vi "Actor Core.vi"(8 "Error In":errorcluster, 11 "KIT-QVG.lvclass":refnum<class "KIT-QVG.lvclass">) -> (0 "Error Out":errorcluster, 3 "Actor out":refnum<class "Actor.lvclass">)   [LabVIEW 2014, in "KIT-QVG.lvlib" / "KIT-QVG.lvclass"]
doc: "(<B>Filename</B>: Actor Framework.lvlib:Actor.lvclass:Actor Core.vi)\n\nReceives messages to the actor, reacts to them, and initiates any error handling that may shut the actor down.\n\nDescendant classes may override this VI to append parallel tasks for the actor to complete while it handles messages. Overrides use the Call Parent Method node."
uses:
  KIT-QVG.lvclass
  <vilib>/ActorFramework/Actor/Actor.lvclass
  CSPP_Core/Actors/CS++BaseActor/CS++BaseActor.lvclass/CS++BaseActor.ctl
  CSPP_Core/Actors/CS++GUIActor/CS++GUIActor.lvclass/CS++GUIActor.ctl
  CSPP_Core/Classes/CS++ProcessVariables/ProcessVariable/PV.lvclass/PV.ctl
  CSPP_Core/Classes/CS++ProcessVariables/PVConnection/PVConnection.lvclass/PVConnection.ctl
  <vilib>/ActorFramework/Actor/Actor.lvclass/Actor.ctl
  <vilib>/ActorFramework/Message Enqueuer/Message Enqueuer.lvclass/Message Enqueuer.ctl
  CSPP_Core/Actors/CS++BaseActor/Read Object Name.vi
  CSPP_Core/Actors/CS++BaseActor/Read CS++Factory.vi
  CSPP_Core/Actors/CS++GUIActor/Read Associated Actor Name.vi
  CSPP_Core/Actors/CS++GUIActor/Read Associated Proxy Actor Name.vi
  CSPP_Core/Classes/CS++ProcessVariables/ProcessVariable/Read Name.vi
  CSPP_Core/Classes/CS++ProcessVariables/ProcessVariable/Read Timestamp.vi
  CSPP_Core/Actors/CS++GUIActor/Read Stop-Event.vi
  CSPP_Core/Actors/CS++GUIActor/Read PV-Update.vi
  <vilib>/ActorFramework/Message Enqueuer/Init from Existing Queue.vi
  <vilib>/ActorFramework/Message Enqueuer/Enqueue.vi
  <vilib>/ActorFramework/Message Priority Queue/Priority Enqueue.vi
  CSPP_Core/Classes/CS++ProcessVariables/PVConnection/PVConnection.lvclass
  CSPP_Core/Classes/CS++BaseClasses/Factory/CS++Factory.lvclass
  CSPP_Core/Classes/CS++ProcessVariables/ProcessVariable/PV.lvclass
  <vilib>/ActorFramework/Message Enqueuer/Message Enqueuer.lvclass
  <vilib>/ActorFramework/Stop Msg/Stop Msg.lvclass
  CSPP_Core/Actors/CS++DeviceGUIActor/CS++DeviceGUIActor.lvclass
  CSPP_Core/Actors/CS++BaseActor/CS++BaseActor.lvclass
  CSPP_Core/Actors/CS++GUIActor/CS++GUIActor.lvclass
  CSPP_Core/Libraries/Utilities/CS++Utilities.lvlib
  CSPP_Core/Classes/CS++ProcessVariables/CS++ProcessVariables.lvlib
panel:
  out "Voltage":dbl[unit][](array[numeric]) format="%.4f"
  out "ADC Raw":i16[](array[numeric])
  out "Hardware Status":T1(array[cluster])
  out "Detector Status":T2(array[cluster])
  out "Temperature":dbl[unit]=273.15
  out "Rack Status":T3
  in  "Detector":u8
  in  "Mute":bool
  in  "Auto Mute":bool
  in  "Mute All":bool
  in  "Quench":bool
  in  "FQuit":bool
  in  "Stop":bool
  in  "Start":bool
  out "Associated Proxy Actor":string
  in  "Stop Button":bool
  out "Timestamp":timestamp
  out "Self-Test Result Message":string
  out "Self-Test Result Code":i32
  out "Resource Name":string
  out "Firmware Revision":string
  out "Driver Revision":string
  out "Associated Worker Actor":string
  # "Resize window to view more details."
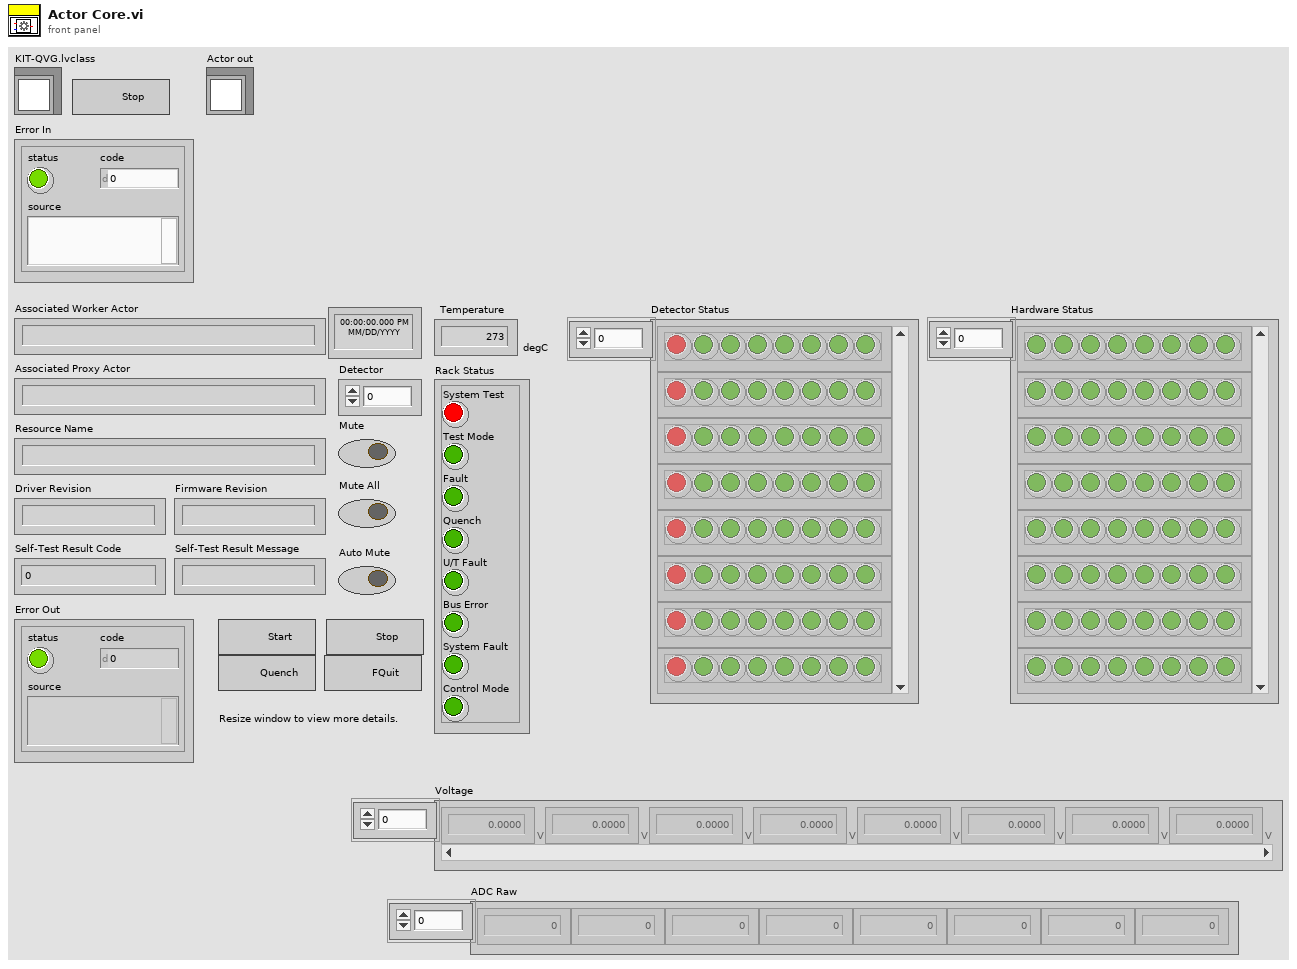
[diagram p1: front panel]
types:
  T1 = cluster{"Q1+":bool, "Q1-":bool, "Q2+":bool, "Q2-":bool, "Mute":bool, "STest-Bit":bool, "QD1":bool, "QD2":bool}[]
  T2 = cluster{"System Test":bool, "Test Mode":bool, "Fault":bool, "Quench":bool, "U/T Fault":bool, "Bus Error":bool, "System Fault":bool, "Reserved":bool}[]
  T3 = cluster{"System Test":bool, "Test Mode":bool, "Fault":bool, "Quench":bool, "U/T Fault":bool, "Bus Error":bool, "System Fault":bool, "Control Mode":bool}
  T4 = cluster{"Read Access":enum8{"Allowed", "Required", "None"}, "Write Access":enum8{"Allowed", "Required", "None"}}
  T5 = enum32{"Invalid", "Standard", "Closed", "Hidden", "Minimized", "Maximized"}
  T6 = cluster{"Q1+":bool, "Q1-":bool, "Q2+":bool, "Q2-":bool, "Mute":bool, "STest-Bit":bool, "QD1":bool, "QD2":bool}
  T7 = cluster{"System Test":bool, "Test Mode":bool, "Fault":bool, "Quench":bool, "U/T Fault":bool, "Bus Error":bool, "System Fault":bool, "Reserved":bool}
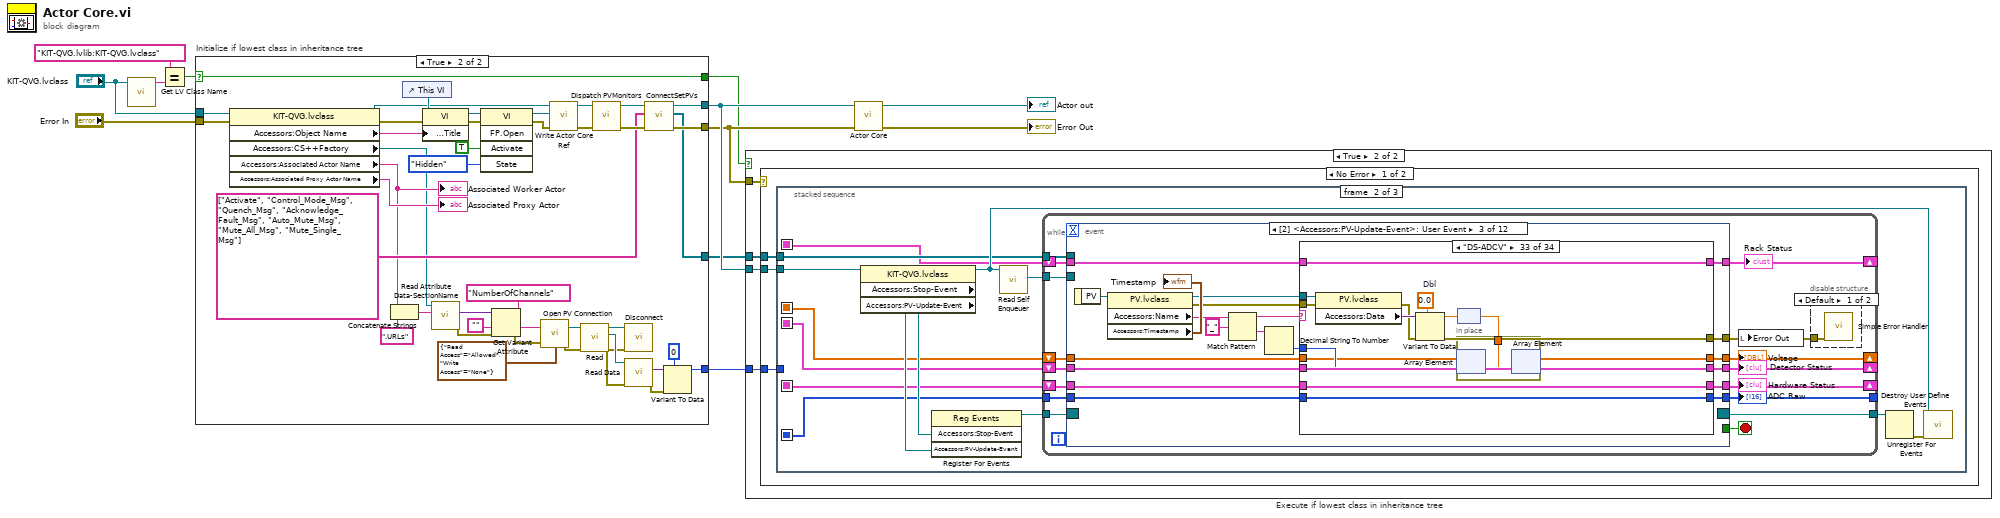
[diagram p0: block diagram]
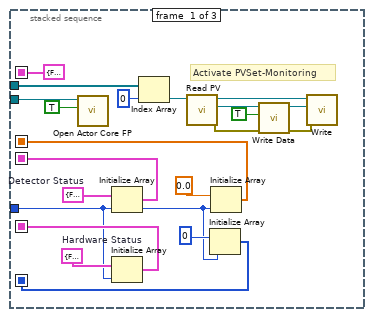
[diagram p3: hidden frame]
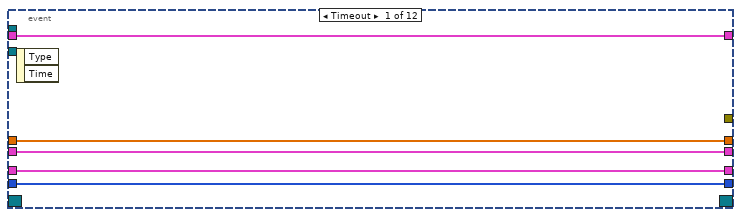
[diagram p5: hidden frame]
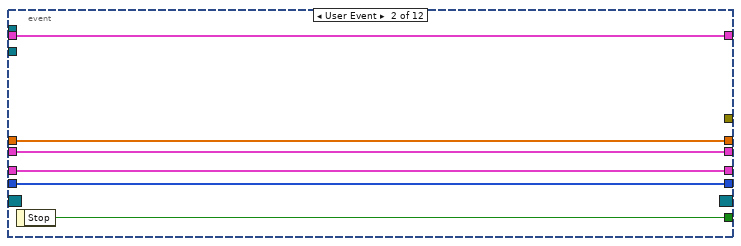
[diagram p6: hidden frame]
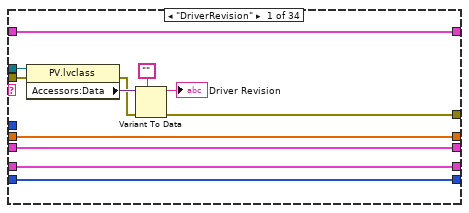
[diagram p7: hidden frame]
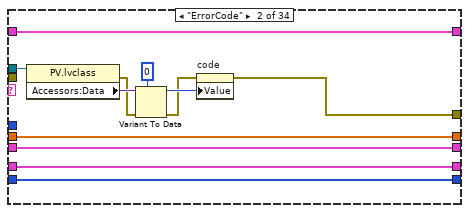
[diagram p8: hidden frame]
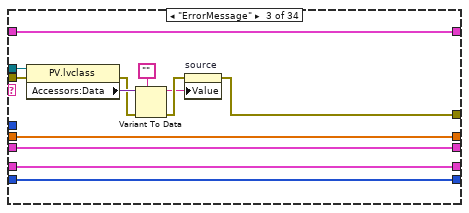
[diagram p9: hidden frame]
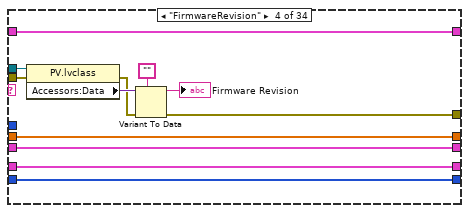
[diagram p10: hidden frame]
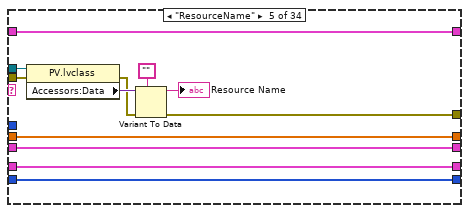
[diagram p11: hidden frame]
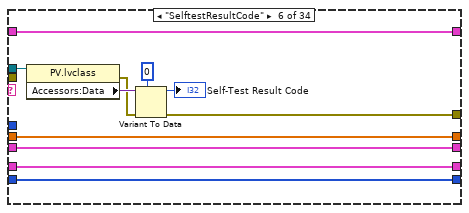
[diagram p12: hidden frame]
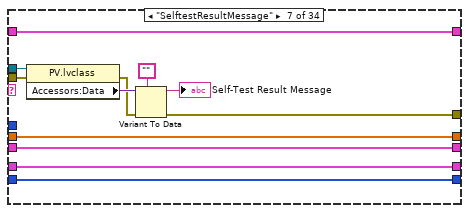
[diagram p13: hidden frame]
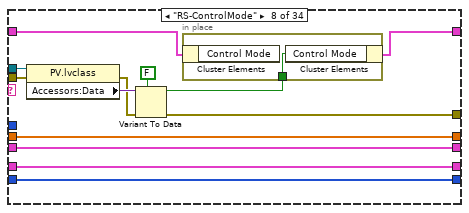
[diagram p14: hidden frame]
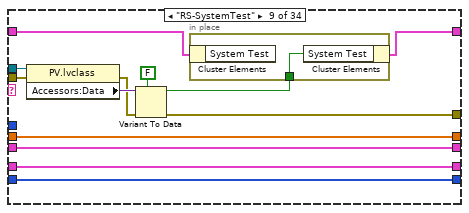
[diagram p15: hidden frame]
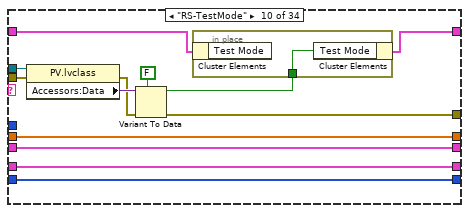
[diagram p16: hidden frame]
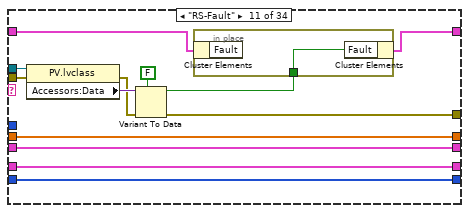
[diagram p17: hidden frame]
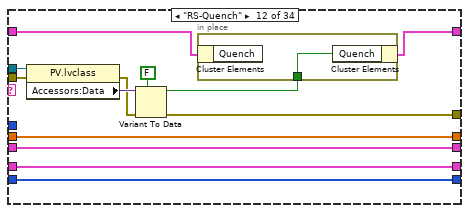
[diagram p18: hidden frame]
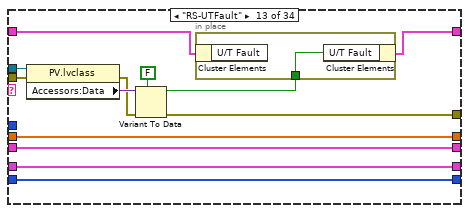
[diagram p19: hidden frame]
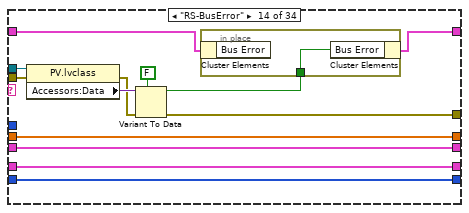
[diagram p20: hidden frame]
diagram:
  n1 = call <vilib>:"Get LV Class Name.vi"("object"="KIT-QVG.lvclass") -> ("class name"=w12:string)  [unwired: 9 in, 1 out]
  n2 = Equal?(x="KIT-QVG.lvlib:KIT-QVG.lvclass" ("class name"), y=w12) -> (x = y?=w9:bool)
  n3 = case "Initialize if lowest class in inheritance tree" shown="True" w9 {
    selector: w9 -> [w15 w55]
    tunnel: "Error In" -> [w13 w46]
    tunnel: "KIT-QVG.lvclass" -> [w14 w53]
    tunnel: [w14 w40] -> w11
    tunnel: [w13 w38] -> w10
    tunnel: [w15 w55] -> w8
    tunnel: [_ w36] -> w2
    tunnel: [_ w16] -> w1
    frame False {
    }
    frame True {
      n4 = property class="KIT-QVG.lvclass"(reference=w53, error in=w46) -> (reference out=w47:refnum<class "KIT-QVG.lvclass">, error out=w48:errorcluster, "Accessors:Object Name"=w45:string, "Accessors:CS++Factory"=w32:refnum<class "CS++Factory.lvclass">, "Accessors:Associated Actor Name"=w33:string, "Accessors:Associated Proxy Actor Name"=→"Associated Proxy Actor":string)
      "Associated Worker Actor" <- w33
      n5 = Concatenate Strings(w33, ".URLs" ("string")) -> (w34:string)
      n6 = control-ref of="This VI"() -> (w51:refnum<vi>)
      n7 = property class="VI"(reference=w51, error in=w48, "Front Panel.Title"=w45) -> (reference out=w50:refnum<vi>, error out=w49:errorcluster)
      n8 = call-dynamic "Read Attribute Data-SectionName.vi"("Object Name"=w34, "CS++Factory in"=w32) -> ("error out"=w30:errorcluster, "Attribute Data"=w31:variant)  [unwired: 7 in, 1 out]
      n9 = invoke class="VI" method="FP.Open"(reference=w50, error in=w49, "Activate"=TRUE ("Activate?"), "State"=T5."Hidden") -> (reference out=w54:refnum<vi>, error out=w52:errorcluster)  [unwired: 1 in, 3 out]
      n10 = Get Variant Attribute(Variant=w31, name="NumberOfChannels", default value (empty Variant)="", error in=w30) -> (value=w27:string, error out=w26:errorcluster)  [unwired: 2 out]
      n11 = call "Open PV Connection.vi"("PV URL"=w27, "Access (R/W allowed)"=T4 {"Read Access"=enum."Allowed", "Write Access"=enum."None"}, "Error In"=w26) -> ("PVConnection"=w24:refnum<class "PVConnection.lvclass">, "Error Out"=w23:errorcluster)
      n12 = call "Write Actor Core Ref.vi"("error in (no error)"=w52, "Actor Core Ref"=w54, "CS++BaseActor in"=w47) -> ("error out"=w43:errorcluster, "CS++BaseActor out"=w44:refnum<class "KIT-QVG.lvclass">)  [unwired: 7 in]
      n13 = call "Read.vi"("error in (no error)"=w23, "PVConnection in"=w24) -> ("error out"=w20:errorcluster, "PV"=w21:refnum<class "PV.lvclass">, "PVConnection out"=w22:refnum<class "PVConnection.lvclass">)  [unwired: 6 in, 1 out]
      n14 = call "Dispatch PVMonitors.vi"("Error In"=w43, "CS++GUIActor in"=w44) -> ("Error Out"=w39:errorcluster, "CS++GUIActor out"=w41:refnum<class "KIT-QVG.lvclass">)  [unwired: 8 in]
      n15 = call "Disconnect.vi"("error in (no error)"=w20, "PVConnection in"=w22) -> ()  [unwired: 8 in, 2 out]
      n16 = call "Read Data.vi"("error in (no error)"=w20, "PV in"=w21) -> ("error out"=w19:errorcluster, "Data"=w18:variant)  [unwired: 7 in, 1 out]
      n17 = call "ConnectSetPVs.vi"("error in (no error)"=w39, "Set-Messages"=string[] ["Activate", "Control_Mode_Msg", "Quench_Msg", "Acknowledge_Fault_Msg", "Auto_Mute_Msg", "Mute_All_Msg", "Mute_Single_Msg"], "CS++GUIActor in"=w41) -> ("error out"=w38:errorcluster, "PVConnections"=w36:refnum<class "PVConnection.lvclass">[], "CS++GUIActor out"=w40:refnum<class "KIT-QVG.lvclass">)  [unwired: 6 in]
      n18 = Variant To Data(error in=w19, type=0, Variant=w18) -> (data=w16:i32)  [unwired: 1 out]
    }
  }
  n19 = case "Execute if lowest class in inheritance tree" shown="True" w8 {
    tunnel: w11 -> [_ w61]
    tunnel: w10 -> [_ w60]
    tunnel: w2 -> [_ w59]
    tunnel: w1 -> [_ w58]
    frame False {
    }
    frame True {
      n20 = case shown="No Error" w60 {
        tunnel: w61 -> [w64 _]
        tunnel: w59 -> [w63 _]
        tunnel: w58 -> [w62 _]
        frame No Error {
          n21 = stacked-sequence {
            seq-local: [w71 _ _] -> [_ w89 _]
            seq-local: [w72 _ _] -> [_ w90 _]
            seq-local: [T3 {"System Test"=FALSE, "Test Mode"=FALSE, "Fault"=FALSE, "Quench"=FALSE, "U/T Fault"=FALSE, "Bus Error"=FALSE, "System Fault"=FALSE, "Control Mode"=FALSE} ("Rack Status") _ _] -> [_ w88 _]
            seq-local: [w66 _ _] -> [_ w86 _]
            seq-local: [w65 _ _] -> [_ w87 _]
            tunnel: w64 -> [w85 w96 w787]
            tunnel: w63 -> [w76 w91 _]
            tunnel: w62 -> [w67 _ _]
            frame #0 {
              w73 = T6 {"Q1+"=FALSE, "Q1-"=FALSE, "Q2+"=FALSE, "Q2-"=FALSE, "Mute"=FALSE, "STest-Bit"=FALSE, "QD1"=FALSE, "QD2"=FALSE}  # Hardware Status
              w74 = T7 {"System Test"=FALSE, "Test Mode"=FALSE, "Fault"=FALSE, "Quench"=FALSE, "U/T Fault"=FALSE, "Bus Error"=FALSE, "System Fault"=FALSE, "Reserved"=FALSE}  # Detector Status
              # "Activate PVSet-Monitoring"
              n22 = call "Open Actor Core FP.vi"("Open FP (F)"=TRUE, "CS++BaseActor in"=w85) -> ()  [unwired: 8 in, 2 out]
              n23 = Initialize Array(w74, w67) -> (w72:T2)
              n24 = Initialize Array(w73, w67) -> (w71:T1)
              n25 = Index Array(array=w76, index=0) -> (element=w82:refnum<class "PVConnection.lvclass">)
              n26 = call "Read PV.vi"("PVConnection in"=w82) -> ("error out"=w78:errorcluster, "PV"=w80:refnum<class "PV.lvclass">, "PVConnection out"=w81:refnum<class "PVConnection.lvclass">)  [unwired: 8 in]
              n27 = Initialize Array(i16 0 ("ADC Raw"), w67) -> (w66:i16[])
              n28 = Initialize Array(dbl[unit] 0.0 ("Volatage"), w67) -> (w65:dbl[unit][])
              n29 = call "Write Data.vi"("error in (no error)"=w78, "Data"=TRUE ("Start"), "PV in"=w80) -> ("error out"=w75:errorcluster, "PV out"=w79:refnum<class "PV.lvclass">)  [unwired: 7 in]
              n30 = call "Write.vi"("error in (no error)"=w75, "PV"=w79, "PVConnection in"=w81) -> ()  [unwired: 7 in, 2 out]
            }
            frame #1 {
              n31 = property class="KIT-QVG.lvclass"(reference=w96) -> (reference out=w95:refnum<class "KIT-QVG.lvclass">, "Accessors:Stop-Event"=w93:refnum<user-event>, "Accessors:PV-Update-Event"=w92:refnum<user-event>)  [unwired: 1 in, 1 out]
              n32 = register-events(w93, w92) -> (reference out=w94:refnum<event-registration>)  [unwired: 2 in, 1 out]
              n33 = call <vilib>:"Read Self Enqueuer.vi"("Actor"=w95) -> ("Self Enqueuer"=w97:refnum<class "Message Enqueuer.lvclass">)  [unwired: 10 in]
              n34 = while {
                tunnel: w94 -> [w115]
                tunnel: [w113] -> w99
                tunnel: w97 -> [w112]
                tunnel: w91 -> [w111]
                shift-right: [w107] -> _
                shift-left: w90 -> [w109]
                shift-right: [w106] -> _
                shift-left: w89 -> [w108]
                shift-right: [w104] -> _
                shift-left: w88 -> [w105]
                tunnel: w86 -> [w102]
                tunnel: [w101] -> _
                shift-right: [w100] -> _
                shift-left: w87 -> [w103]
                stop <- w114 stop-if-true
                n35 = event shown="[2] <Accessors:PV-Update-Event>: User Event" {
                  selector: w115 -> [_ _ _ _ _ _ _ _ _ _ _ _]
                  dyn-events: [_ _ _ _ _ _ _ _ _ _ _ _] -> w113
                  timeout: _ -> [_ _ _ _ _ _ _ _ _ _ _ _]
                  tunnel: [_ w127 _ _ _ _ _ _ _ _ _ _] -> w114
                  tunnel: [_ _ w143 w670 w676 w684 w699 w714 w729 w745 w760 w777] -> w110
                  tunnel: w112 -> [_ _ _ w669 w677 _ _ _ _ _ _ _]
                  tunnel: w111 -> [_ _ _ _ _ w693 w708 w723 w738 w753 w768 w785]
                  tunnel: w109 -> [w118 w123 w137 w665 w672 w680 w695 w710 w725 w740 w755 w770]
                  tunnel: w108 -> [w120 w125 w136 w667 w674 w682 w697 w712 w727 w742 w757 w772]
                  tunnel: [w118 w123 w135 w665 w672 w680 w695 w710 w725 w740 w755 w770] -> w107
                  tunnel: [w120 w125 w134 w667 w674 w682 w697 w712 w727 w742 w757 w772] -> w106
                  tunnel: w105 -> [w121 w126 w133 w668 w675 w683 w698 w713 w728 w743 w758 w773]
                  tunnel: [w121 w126 w132 w668 w675 w683 w698 w713 w728 w743 w758 w773] -> w104
                  tunnel: w103 -> [w117 w122 w131 w664 w671 w679 w694 w709 w724 w739 w754 w769]
                  tunnel: w102 -> [w119 w124 w130 w666 w673 w681 w696 w711 w726 w741 w756 w771]
                  tunnel: [w119 w124 w129 w666 w673 w681 w696 w711 w726 w741 w756 w771] -> w101
                  tunnel: [w117 w122 w128 w664 w671 w679 w694 w709 w724 w739 w754 w769] -> w100
                  event Timeout {
                    n36 = event-data() -> ()  [unwired: 1 in, 2 out]
                  }
                  event User Event {
                    n37 = event-data() -> ("Stop"=w127:bool)  [unwired: 1 in]
                  }
                  event User Event {
                    n38 = event-data() -> ("PV"=w144:refnum<class "PV.lvclass">)  [unwired: 1 in]
                    n39 = property class="PV.lvclass"(reference=w144) -> (reference out=w145:refnum<class "PV.lvclass">, error out=w146:errorcluster, "Accessors:Name"=w142:string, "Accessors:Timestamp"=→"Timestamp":timestamp)  [unwired: 1 in]
                    n40 = Match Pattern(string=w142, regular expression="_") -> (before substring=w141:string, after substring=w139:string)  [unwired: 1 in, 2 out]
                    n41 = Decimal String To Number(string=w139) -> (number=w138:i32)  [unwired: 2 in, 1 out]
                    n42 = case shown="\"DS-ADCV\"" w141 {
                      tunnel: w145 -> [w157 w169 w182 w194 w206 w217 w229 w243 w257 w271 w285 w299 w313 w327 w341 w355 w369 w387 w405 w423 w441 w459 w477 w495 w513 w531 w549 w567 w585 w603 w621 w639 w655 _]
                      tunnel: w146 -> [w156 _ w181 w193 w205 _ w228 w242 w256 w270 w284 w298 w312 w326 w340 w354 w368 w386 w404 w422 w440 w458 w476 w494 w512 w530 w548 w566 w584 w602 w620 w638 w654 w663]
                      tunnel: [w153 w165 w178 w190 w202 w215 w225 w237 w251 w265 w279 w293 w307 w321 w334 w349 w365 w383 w401 w419 w437 w455 w473 w491 w509 w527 w545 w563 w581 w599 w617 w635 w651 w663] -> w143
                      tunnel: w138 -> [_ _ _ _ _ _ _ _ _ _ _ _ _ _ _ _ w359 w377 w395 w413 w431 w449 w467 w485 w503 w521 w539 w557 w575 w593 w611 w629 w647 _]
                      tunnel: w137 -> [w151 w163 w175 w188 w200 w212 w223 w238 w252 w266 w280 w294 w308 w322 w336 w347 w364 w382 w400 w418 w436 w454 w472 w487 w505 w523 w541 w559 w577 w595 w613 w634 w650 w661]
                      tunnel: w136 -> [w152 w164 w176 w189 w201 w213 w224 w239 w253 w267 w281 w295 w309 w323 w337 w348 w362 w380 w398 w416 w434 w452 w470 w489 w507 w525 w543 w561 w579 w597 w615 w628 w646 w662]
                      tunnel: [w151 w163 w175 w188 w200 w212 w223 w238 w252 w266 w280 w294 w308 w322 w336 w347 w363 w381 w399 w417 w435 w453 w471 w487 w505 w523 w541 w559 w577 w595 w613 w634 w650 w661] -> w135
                      tunnel: [w152 w164 w176 w189 w201 w213 w224 w239 w253 w267 w281 w295 w309 w323 w337 w348 w362 w380 w398 w416 w434 w452 w470 w488 w506 w524 w542 w560 w578 w596 w614 w628 w646 w662] -> w134
                      tunnel: w133 -> [w150 w162 w174 w187 w199 w211 w222 w236 w250 w264 w278 w292 w306 w320 w335 w346 w360 w378 w396 w414 w432 w450 w468 w486 w504 w522 w540 w558 w576 w594 w612 w633 w649 w660]
                      tunnel: [w150 w162 w174 w187 w199 w211 w222 w235 w249 w263 w277 w291 w305 w319 w332 w346 w360 w378 w396 w414 w432 w450 w468 w486 w504 w522 w540 w558 w576 w594 w612 w633 w649 w660] -> w132
                      tunnel: w131 -> [w149 w161 w173 w186 w198 w210 w221 w233 w247 w261 w275 w289 w303 w317 w331 w345 w358 w376 w394 w412 w430 w448 w466 w484 w502 w520 w538 w556 w574 w592 w610 w627 w645 w659]
                      tunnel: w130 -> [w148 w160 w172 w185 w197 w209 w220 w232 w246 w260 w274 w288 w302 w316 w330 w344 w357 w375 w393 w411 w429 w447 w465 w483 w501 w519 w537 w555 w573 w591 w609 w632 w642 w658]
                      tunnel: [w148 w160 w172 w185 w197 w209 w220 w232 w246 w260 w274 w288 w302 w316 w330 w344 w357 w375 w393 w411 w429 w447 w465 w483 w501 w519 w537 w555 w573 w591 w609 w630 w642 w658] -> w129
                      tunnel: [w149 w161 w173 w186 w198 w210 w221 w233 w247 w261 w275 w289 w303 w317 w331 w345 w358 w376 w394 w412 w430 w448 w466 w484 w502 w520 w538 w556 w574 w592 w610 w627 w644 w659] -> w128
                      frame "DriverRevision" {
                        n43 = property class="PV.lvclass"(reference=w157, error in=w156) -> (error out=w155:errorcluster, "Accessors:Data"=w158:variant)  [unwired: 1 out]
                        n44 = Variant To Data(error in=w155, type="", Variant=w158) -> (data=→"Driver Revision":string, error out=w153:errorcluster)
                      }
                      frame "ErrorCode" {
                        n45 = property class="PV.lvclass"(reference=w169) -> (error out=w168:errorcluster, "Accessors:Data"=w170:variant)  [unwired: 1 in, 1 out]
                        n46 = Variant To Data(error in=w168, type=0, Variant=w170) -> (data=w167:i32, error out=w166:errorcluster)
                        n47 = property on="code" class="DigNum (strict)"(error in=w166, "Value"=w167) -> (error out=w165:errorcluster)  [unwired: 1 in, 1 out]
                      }
                      frame "ErrorMessage" {
                        n48 = property class="PV.lvclass"(reference=w182, error in=w181) -> (error out=w180:errorcluster, "Accessors:Data"=w183:variant)  [unwired: 1 out]
                        n49 = Variant To Data(error in=w180, type="", Variant=w183) -> (data=w177:string, error out=w179:errorcluster)
                        n50 = property on="source" class="Str"(error in=w179, "Value"=w177) -> (error out=w178:errorcluster)  [unwired: 1 in, 1 out]
                      }
                      frame "FirmwareRevision" {
                        n51 = property class="PV.lvclass"(reference=w194, error in=w193) -> (error out=w192:errorcluster, "Accessors:Data"=w195:variant)  [unwired: 1 out]
                        n52 = Variant To Data(error in=w192, type="", Variant=w195) -> (data=→"Firmware Revision":string, error out=w190:errorcluster)
                      }
                      frame "ResourceName" {
                        n53 = property class="PV.lvclass"(reference=w206, error in=w205) -> (error out=w204:errorcluster, "Accessors:Data"=w207:variant)  [unwired: 1 out]
                        n54 = Variant To Data(error in=w204, type="", Variant=w207) -> (data=→"Resource Name":string, error out=w202:errorcluster)
                      }
                      frame "SelftestResultCode" {
                        n55 = property class="PV.lvclass"(reference=w217) -> (error out=w214:errorcluster, "Accessors:Data"=w218:variant)  [unwired: 1 in, 1 out]
                        n56 = Variant To Data(error in=w214, type=0, Variant=w218) -> (data=→"Self-Test Result Code":i32, error out=w215:errorcluster)
                      }
                      frame "SelftestResultMessage" {
                        n57 = property class="PV.lvclass"(reference=w229, error in=w228) -> (error out=w227:errorcluster, "Accessors:Data"=w230:variant)  [unwired: 1 out]
                        n58 = Variant To Data(error in=w227, type="", Variant=w230) -> (data=→"Self-Test Result Message":string, error out=w225:errorcluster)
                      }
                      frame "RS-ControlMode" {
                        n59 = property class="PV.lvclass"(reference=w243, error in=w242) -> (error out=w241:errorcluster, "Accessors:Data"=w244:variant)  [unwired: 1 out]
                        n60 = Variant To Data(error in=w241, type=FALSE ("Value"), Variant=w244) -> (data=w234:bool, error out=w237:errorcluster)
                        n61 = in-place {
                          in-place-border: w234 -> [w245]
                          n62 = in-place-cluster #1(w236) -> ()  [unwired: 1 out]
                          n63 = in-place-cluster #1("Control Mode"=w245) -> (w235:T3)
                        }
                      }
                      frame "RS-SystemTest" {
                        n64 = property class="PV.lvclass"(reference=w257, error in=w256) -> (error out=w255:errorcluster, "Accessors:Data"=w258:variant)  [unwired: 1 out]
                        n65 = Variant To Data(error in=w255, type=FALSE ("Value"), Variant=w258) -> (data=w248:bool, error out=w251:errorcluster)
                        n66 = in-place {
                          in-place-border: w248 -> [w259]
                          n67 = in-place-cluster #2(w250) -> ()  [unwired: 1 out]
                          n68 = in-place-cluster #2("System Test"=w259) -> (w249:T3)
                        }
                      }
                      frame "RS-TestMode" {
                        n69 = property class="PV.lvclass"(reference=w271, error in=w270) -> (error out=w269:errorcluster, "Accessors:Data"=w272:variant)  [unwired: 1 out]
                        n70 = Variant To Data(error in=w269, type=FALSE ("Value"), Variant=w272) -> (data=w262:bool, error out=w265:errorcluster)
                        n71 = in-place {
                          in-place-border: w262 -> [w273]
                          n72 = in-place-cluster #3(w264) -> ()  [unwired: 1 out]
                          n73 = in-place-cluster #3("Test Mode"=w273) -> (w263:T3)
                        }
                      }
                      frame "RS-Fault" {
                        n74 = property class="PV.lvclass"(reference=w285, error in=w284) -> (error out=w283:errorcluster, "Accessors:Data"=w286:variant)  [unwired: 1 out]
                        n75 = Variant To Data(error in=w283, type=FALSE ("Value"), Variant=w286) -> (data=w276:bool, error out=w279:errorcluster)
                        n76 = in-place {
                          in-place-border: w276 -> [w287]
                          n77 = in-place-cluster #4(w278) -> ()  [unwired: 1 out]
                          n78 = in-place-cluster #4("Fault"=w287) -> (w277:T3)
                        }
                      }
                      frame "RS-Quench" {
                        n79 = property class="PV.lvclass"(reference=w299, error in=w298) -> (error out=w297:errorcluster, "Accessors:Data"=w300:variant)  [unwired: 1 out]
                        n80 = Variant To Data(error in=w297, type=FALSE ("Value"), Variant=w300) -> (data=w290:bool, error out=w293:errorcluster)
                        n81 = in-place {
                          in-place-border: w290 -> [w301]
                          n82 = in-place-cluster #5(w292) -> ()  [unwired: 1 out]
                          n83 = in-place-cluster #5("Quench"=w301) -> (w291:T3)
                        }
                      }
                      frame "RS-UTFault" {
                        n84 = property class="PV.lvclass"(reference=w313, error in=w312) -> (error out=w311:errorcluster, "Accessors:Data"=w314:variant)  [unwired: 1 out]
                        n85 = Variant To Data(error in=w311, type=FALSE ("Value"), Variant=w314) -> (data=w304:bool, error out=w307:errorcluster)
                        n86 = in-place {
                          in-place-border: w304 -> [w315]
                          n87 = in-place-cluster #6(w306) -> ()  [unwired: 1 out]
                          n88 = in-place-cluster #6("U/T Fault"=w315) -> (w305:T3)
                        }
                      }
                      frame "RS-BusError" {
                        n89 = property class="PV.lvclass"(reference=w327, error in=w326) -> (error out=w325:errorcluster, "Accessors:Data"=w328:variant)  [unwired: 1 out]
                        n90 = Variant To Data(error in=w325, type=FALSE ("Value"), Variant=w328) -> (data=w318:bool, error out=w321:errorcluster)
                        n91 = in-place {
                          in-place-border: w318 -> [w329]
                          n92 = in-place-cluster #7(w320) -> ()  [unwired: 1 out]
                          n93 = in-place-cluster #7("Bus Error"=w329) -> (w319:T3)
                        }
                      }
                      frame "RS-SystemFault" {
                        n94 = property class="PV.lvclass"(reference=w341, error in=w340) -> (error out=w339:errorcluster, "Accessors:Data"=w342:variant)  [unwired: 1 out]
                        n95 = Variant To Data(error in=w339, type=FALSE ("Value"), Variant=w342) -> (data=w333:bool, error out=w334:errorcluster)
                        n96 = in-place {
                          in-place-border: w333 -> [w343]
                          n97 = in-place-cluster #8(w335) -> ()  [unwired: 1 out]
                          n98 = in-place-cluster #8("System Fault"=w343) -> (w332:T3)
                        }
                      }
                      frame "RS-AveragedT" {
                        n99 = property class="PV.lvclass"(reference=w355, error in=w354) -> (error out=w353:errorcluster, "Accessors:Data"=w356:variant)  [unwired: 1 out]
                        n100 = Variant To Data(error in=w353, type=0.0 ("Value"), Variant=w356) -> (data=w351:dbl, error out=w349:errorcluster)
                        n101 = node(w351) -> (→"Temperature":dbl[unit])
                      }
                      frame "DS-SystemTest" {
                        n102 = property class="PV.lvclass"(reference=w369, error in=w368) -> (error out=w367:errorcluster, "Accessors:Data"=w370:variant)  [unwired: 1 out]
                        n103 = Variant To Data(error in=w367, type=FALSE, Variant=w370) -> (data=w361:bool, error out=w365:errorcluster)
                        n104 = in-place {
                          in-place-border: w361 -> [w371]
                          n105 = in-place-array #9(w364, w359) -> (w373:T7)
                          n106 = in-place {
                            in-place-border: w371 -> [w374]
                            n107 = in-place-cluster #10(w373) -> ()  [unwired: 1 out]
                            n108 = in-place-cluster #10("System Test"=w374) -> (w372:T7)
                          }
                          n109 = in-place-array #9(w372) -> (w363:T2)  [unwired: 1 out]
                        }
                      }
                      frame "DS-TestMode" {
                        n110 = property class="PV.lvclass"(reference=w387, error in=w386) -> (error out=w385:errorcluster, "Accessors:Data"=w388:variant)  [unwired: 1 out]
                        n111 = Variant To Data(error in=w385, type=FALSE, Variant=w388) -> (data=w379:bool, error out=w383:errorcluster)
                        n112 = in-place {
                          in-place-border: w379 -> [w389]
                          n113 = in-place-array #11(w382, w377) -> (w391:T7)
                          n114 = in-place {
                            in-place-border: w389 -> [w392]
                            n115 = in-place-cluster #12(w391) -> ()  [unwired: 1 out]
                            n116 = in-place-cluster #12("Test Mode"=w392) -> (w390:T7)
                          }
                          n117 = in-place-array #11(w390) -> (w381:T2)  [unwired: 1 out]
                        }
                      }
                      frame "DS-Fault" {
                        n118 = property class="PV.lvclass"(reference=w405, error in=w404) -> (error out=w403:errorcluster, "Accessors:Data"=w406:variant)  [unwired: 1 out]
                        n119 = Variant To Data(error in=w403, type=FALSE, Variant=w406) -> (data=w397:bool, error out=w401:errorcluster)
                        n120 = in-place {
                          in-place-border: w397 -> [w407]
                          n121 = in-place-array #13(w400, w395) -> (w409:T7)
                          n122 = in-place {
                            in-place-border: w407 -> [w410]
                            n123 = in-place-cluster #14(w409) -> ()  [unwired: 1 out]
                            n124 = in-place-cluster #14("Fault"=w410) -> (w408:T7)
                          }
                          n125 = in-place-array #13(w408) -> (w399:T2)  [unwired: 1 out]
                        }
                      }
                      frame "DS-Quench" {
                        n126 = property class="PV.lvclass"(reference=w423, error in=w422) -> (error out=w421:errorcluster, "Accessors:Data"=w424:variant)  [unwired: 1 out]
                        n127 = Variant To Data(error in=w421, type=FALSE, Variant=w424) -> (data=w415:bool, error out=w419:errorcluster)
                        n128 = in-place {
                          in-place-border: w415 -> [w425]
                          n129 = in-place-array #15(w418, w413) -> (w427:T7)
                          n130 = in-place {
                            in-place-border: w425 -> [w428]
                            n131 = in-place-cluster #16(w427) -> ()  [unwired: 1 out]
                            n132 = in-place-cluster #16("Quench"=w428) -> (w426:T7)
                          }
                          n133 = in-place-array #15(w426) -> (w417:T2)  [unwired: 1 out]
                        }
                      }
                      frame "DS-UTFault" {
                        n134 = property class="PV.lvclass"(reference=w441, error in=w440) -> (error out=w439:errorcluster, "Accessors:Data"=w442:variant)  [unwired: 1 out]
                        n135 = Variant To Data(error in=w439, type=FALSE, Variant=w442) -> (data=w433:bool, error out=w437:errorcluster)
                        n136 = in-place {
                          in-place-border: w433 -> [w443]
                          n137 = in-place-array #17(w436, w431) -> (w445:T7)
                          n138 = in-place {
                            in-place-border: w443 -> [w446]
                            n139 = in-place-cluster #18(w445) -> ()  [unwired: 1 out]
                            n140 = in-place-cluster #18("U/T Fault"=w446) -> (w444:T7)
                          }
                          n141 = in-place-array #17(w444) -> (w435:T2)  [unwired: 1 out]
                        }
                      }
                      frame "DS-BusError" {
                        n142 = property class="PV.lvclass"(reference=w459, error in=w458) -> (error out=w457:errorcluster, "Accessors:Data"=w460:variant)  [unwired: 1 out]
                        n143 = Variant To Data(error in=w457, type=FALSE, Variant=w460) -> (data=w451:bool, error out=w455:errorcluster)
                        n144 = in-place {
                          in-place-border: w451 -> [w461]
                          n145 = in-place-array #19(w454, w449) -> (w463:T7)
                          n146 = in-place {
                            in-place-border: w461 -> [w464]
                            n147 = in-place-cluster #20(w463) -> ()  [unwired: 1 out]
                            n148 = in-place-cluster #20("Bus Error"=w464) -> (w462:T7)
                          }
                          n149 = in-place-array #19(w462) -> (w453:T2)  [unwired: 1 out]
                        }
                      }
                      frame "DS-SystemFault" {
                        n150 = property class="PV.lvclass"(reference=w477, error in=w476) -> (error out=w475:errorcluster, "Accessors:Data"=w478:variant)  [unwired: 1 out]
                        n151 = Variant To Data(error in=w475, type=FALSE, Variant=w478) -> (data=w469:bool, error out=w473:errorcluster)
                        n152 = in-place {
                          in-place-border: w469 -> [w479]
                          n153 = in-place-array #21(w472, w467) -> (w481:T7)
                          n154 = in-place {
                            in-place-border: w479 -> [w482]
                            n155 = in-place-cluster #22(w481) -> ()  [unwired: 1 out]
                            n156 = in-place-cluster #22("System Fault"=w482) -> (w480:T7)
                          }
                          n157 = in-place-array #21(w480) -> (w471:T2)  [unwired: 1 out]
                        }
                      }
                      frame "HW-Q1P" {
                        n158 = property class="PV.lvclass"(reference=w495, error in=w494) -> (error out=w493:errorcluster, "Accessors:Data"=w496:variant)  [unwired: 1 out]
                        n159 = Variant To Data(error in=w493, type=FALSE, Variant=w496) -> (data=w490:bool, error out=w491:errorcluster)
                        n160 = in-place {
                          in-place-border: w490 -> [w497]
                          n161 = in-place-array #23(w489, w485) -> (w499:T6)
                          n162 = in-place {
                            in-place-border: w497 -> [w500]
                            n163 = in-place-cluster #24(w499) -> ()  [unwired: 1 out]
                            n164 = in-place-cluster #24("Q1+"=w500) -> (w498:T6)
                          }
                          n165 = in-place-array #23(w498) -> (w488:T1)  [unwired: 1 out]
                        }
                      }
                      frame "HW-Q1M" {
                        n166 = property class="PV.lvclass"(reference=w513, error in=w512) -> (error out=w511:errorcluster, "Accessors:Data"=w514:variant)  [unwired: 1 out]
                        n167 = Variant To Data(error in=w511, type=FALSE, Variant=w514) -> (data=w508:bool, error out=w509:errorcluster)
                        n168 = in-place {
                          in-place-border: w508 -> [w515]
                          n169 = in-place-array #25(w507, w503) -> (w517:T6)
                          n170 = in-place {
                            in-place-border: w515 -> [w518]
                            n171 = in-place-cluster #26(w517) -> ()  [unwired: 1 out]
                            n172 = in-place-cluster #26("Q1-"=w518) -> (w516:T6)
                          }
                          n173 = in-place-array #25(w516) -> (w506:T1)  [unwired: 1 out]
                        }
                      }
                      frame "HW-Q2P" {
                        n174 = property class="PV.lvclass"(reference=w531, error in=w530) -> (error out=w529:errorcluster, "Accessors:Data"=w532:variant)  [unwired: 1 out]
                        n175 = Variant To Data(error in=w529, type=FALSE, Variant=w532) -> (data=w526:bool, error out=w527:errorcluster)
                        n176 = in-place {
                          in-place-border: w526 -> [w533]
                          n177 = in-place-array #27(w525, w521) -> (w535:T6)
                          n178 = in-place {
                            in-place-border: w533 -> [w536]
                            n179 = in-place-cluster #28(w535) -> ()  [unwired: 1 out]
                            n180 = in-place-cluster #28("Q2+"=w536) -> (w534:T6)
                          }
                          n181 = in-place-array #27(w534) -> (w524:T1)  [unwired: 1 out]
                        }
                      }
                      frame "HW-Q2M" {
                        n182 = property class="PV.lvclass"(reference=w549, error in=w548) -> (error out=w547:errorcluster, "Accessors:Data"=w550:variant)  [unwired: 1 out]
                        n183 = Variant To Data(error in=w547, type=FALSE, Variant=w550) -> (data=w544:bool, error out=w545:errorcluster)
                        n184 = in-place {
                          in-place-border: w544 -> [w551]
                          n185 = in-place-array #29(w543, w539) -> (w553:T6)
                          n186 = in-place {
                            in-place-border: w551 -> [w554]
                            n187 = in-place-cluster #30(w553) -> ()  [unwired: 1 out]
                            n188 = in-place-cluster #30("Q2-"=w554) -> (w552:T6)
                          }
                          n189 = in-place-array #29(w552) -> (w542:T1)  [unwired: 1 out]
                        }
                      }
                      frame "HW-Mute" {
                        n190 = property class="PV.lvclass"(reference=w567, error in=w566) -> (error out=w565:errorcluster, "Accessors:Data"=w568:variant)  [unwired: 1 out]
                        n191 = Variant To Data(error in=w565, type=FALSE, Variant=w568) -> (data=w562:bool, error out=w563:errorcluster)
                        n192 = in-place {
                          in-place-border: w562 -> [w569]
                          n193 = in-place-array #31(w561, w557) -> (w571:T6)
                          n194 = in-place {
                            in-place-border: w569 -> [w572]
                            n195 = in-place-cluster #32(w571) -> ()  [unwired: 1 out]
                            n196 = in-place-cluster #32("Mute"=w572) -> (w570:T6)
                          }
                          n197 = in-place-array #31(w570) -> (w560:T1)  [unwired: 1 out]
                        }
                      }
                      frame "HW-STestBit" {
                        n198 = property class="PV.lvclass"(reference=w585, error in=w584) -> (error out=w583:errorcluster, "Accessors:Data"=w586:variant)  [unwired: 1 out]
                        n199 = Variant To Data(error in=w583, type=FALSE, Variant=w586) -> (data=w580:bool, error out=w581:errorcluster)
                        n200 = in-place {
                          in-place-border: w580 -> [w587]
                          n201 = in-place-array #33(w579, w575) -> (w589:T6)
                          n202 = in-place {
                            in-place-border: w587 -> [w590]
                            n203 = in-place-cluster #34(w589) -> ()  [unwired: 1 out]
                            n204 = in-place-cluster #34("STest-Bit"=w590) -> (w588:T6)
                          }
                          n205 = in-place-array #33(w588) -> (w578:T1)  [unwired: 1 out]
                        }
                      }
                      frame "HW-QD1" {
                        n206 = property class="PV.lvclass"(reference=w603, error in=w602) -> (error out=w601:errorcluster, "Accessors:Data"=w604:variant)  [unwired: 1 out]
                        n207 = Variant To Data(error in=w601, type=FALSE, Variant=w604) -> (data=w598:bool, error out=w599:errorcluster)
                        n208 = in-place {
                          in-place-border: w598 -> [w605]
                          n209 = in-place-array #35(w597, w593) -> (w607:T6)
                          n210 = in-place {
                            in-place-border: w605 -> [w608]
                            n211 = in-place-cluster #36(w607) -> ()  [unwired: 1 out]
                            n212 = in-place-cluster #36("QD1"=w608) -> (w606:T6)
                          }
                          n213 = in-place-array #35(w606) -> (w596:T1)  [unwired: 1 out]
                        }
                      }
                      frame "HW-QD2" {
                        n214 = property class="PV.lvclass"(reference=w621, error in=w620) -> (error out=w619:errorcluster, "Accessors:Data"=w622:variant)  [unwired: 1 out]
                        n215 = Variant To Data(error in=w619, type=FALSE, Variant=w622) -> (data=w616:bool, error out=w617:errorcluster)
                        n216 = in-place {
                          in-place-border: w616 -> [w623]
                          n217 = in-place-array #37(w615, w611) -> (w625:T6)
                          n218 = in-place {
                            in-place-border: w623 -> [w626]
                            n219 = in-place-cluster #38(w625) -> ()  [unwired: 1 out]
                            n220 = in-place-cluster #38("QD2"=w626) -> (w624:T6)
                          }
                          n221 = in-place-array #37(w624) -> (w614:T1)  [unwired: 1 out]
                        }
                      }
                      frame "DS-ADCRaw" {
                        w636 = i16 0  # I16
                        n222 = property class="PV.lvclass"(reference=w639, error in=w638) -> (error out=w637:errorcluster, "Accessors:Data"=w640:variant)  [unwired: 1 out]
                        n223 = Variant To Data(error in=w637, type=w636, Variant=w640) -> (data=w631:i16, error out=w635:errorcluster)
                        n224 = in-place {
                          in-place-border: w631 -> [w641]
                          n225 = in-place-array #39(w632, w629) -> ()  [unwired: 1 out]
                          n226 = in-place-array #39(w641) -> (w630:i16[])  [unwired: 1 out]
                        }
                      }
                      frame "DS-ADCV" {
                        w652 = 0.0  # Dbl
                        n227 = property class="PV.lvclass"(reference=w655, error in=w654) -> (error out=w653:errorcluster, "Accessors:Data"=w656:variant)  [unwired: 1 out]
                        n228 = Variant To Data(error in=w653, type=w652, Variant=w656) -> (data=w648:dbl, error out=w651:errorcluster)
                        n229 = node(w648) -> (w643:dbl[unit])
                        n230 = in-place {
                          in-place-border: w643 -> [w657]
                          n231 = in-place-array #40(w645, w647) -> ()  [unwired: 1 out]
                          n232 = in-place-array #40(w657) -> (w644:dbl[unit][])  [unwired: 1 out]
                        }
                      }
                      frame Default {
                      }
                    }
                  }
                  event "Stop Button": Value Change {
                    n233 = event-data() -> ()  [unwired: 1 in, 1 out]
                    n234 = call <vilib>:"Send Normal Stop.vi"("Message Enqueuer"=w669) -> ("error out"=w670:errorcluster)  [unwired: 10 in]
                  }
                  event Panel Close? {
                    n235 = event-data() -> ()  [unwired: 1 in, 1 out]
                    n236 = call "Close Window or Stop Actor Dialog.vi"("Self Enqueuer"=w677) -> ("Error Out"=w676:errorcluster)  [unwired: 2 in]
                    n237 = event-data("Discard?"=TRUE) -> ()  [unwired: 1 in, 1 out]
                  }
                  event "Start": Value Change {
                    n238 = event-data() -> ()  [unwired: 1 in, 1 out]
                    n239 = Index Array(array=w693, index=1) -> (element=w691:refnum<class "PVConnection.lvclass">)
                    n240 = call "Read PV.vi"("PVConnection in"=w691) -> ("error out"=w687:errorcluster, "PV"=w689:refnum<class "PV.lvclass">, "PVConnection out"=w690:refnum<class "PVConnection.lvclass">)  [unwired: 8 in]
                    n241 = call "Write Data.vi"("error in (no error)"=w687, "Data"=TRUE ("Start"), "PV in"=w689) -> ("error out"=w686:errorcluster, "PV out"=w688:refnum<class "PV.lvclass">)  [unwired: 7 in]
                    n242 = call "Write.vi"("error in (no error)"=w686, "PV"=w688, "PVConnection in"=w690) -> ("error out"=w684:errorcluster)  [unwired: 7 in, 1 out]
                  }
                  event "Stop": Value Change {
                    n243 = event-data() -> ()  [unwired: 1 in, 1 out]
                    n244 = Index Array(array=w708, index=1) -> (element=w706:refnum<class "PVConnection.lvclass">)
                    n245 = call "Read PV.vi"("PVConnection in"=w706) -> ("error out"=w702:errorcluster, "PV"=w704:refnum<class "PV.lvclass">, "PVConnection out"=w705:refnum<class "PVConnection.lvclass">)  [unwired: 8 in]
                    n246 = call "Write Data.vi"("error in (no error)"=w702, "Data"=FALSE ("Start"), "PV in"=w704) -> ("error out"=w701:errorcluster, "PV out"=w703:refnum<class "PV.lvclass">)  [unwired: 7 in]
                    n247 = call "Write.vi"("error in (no error)"=w701, "PV"=w703, "PVConnection in"=w705) -> ("error out"=w699:errorcluster)  [unwired: 7 in, 1 out]
                  }
                  event "Quench": Value Change {
                    n248 = event-data() -> ()  [unwired: 1 in, 1 out]
                    n249 = Index Array(array=w723, index=2) -> (element=w721:refnum<class "PVConnection.lvclass">)
                    n250 = call "Read PV.vi"("PVConnection in"=w721) -> ("error out"=w717:errorcluster, "PV"=w719:refnum<class "PV.lvclass">, "PVConnection out"=w720:refnum<class "PVConnection.lvclass">)  [unwired: 8 in]
                    n251 = call "Write Data.vi"("error in (no error)"=w717, "Data"=TRUE ("Start"), "PV in"=w719) -> ("error out"=w716:errorcluster, "PV out"=w718:refnum<class "PV.lvclass">)  [unwired: 7 in]
                    n252 = call "Write.vi"("error in (no error)"=w716, "PV"=w718, "PVConnection in"=w720) -> ("error out"=w714:errorcluster)  [unwired: 7 in, 1 out]
                  }
                  event "FQuit": Value Change {
                    n253 = event-data() -> ()  [unwired: 1 in, 1 out]
                    n254 = Index Array(array=w738, index=3) -> (element=w736:refnum<class "PVConnection.lvclass">)
                    n255 = call "Read PV.vi"("PVConnection in"=w736) -> ("error out"=w732:errorcluster, "PV"=w734:refnum<class "PV.lvclass">, "PVConnection out"=w735:refnum<class "PVConnection.lvclass">)  [unwired: 8 in]
                    n256 = call "Write Data.vi"("error in (no error)"=w732, "Data"=TRUE ("Start"), "PV in"=w734) -> ("error out"=w731:errorcluster, "PV out"=w733:refnum<class "PV.lvclass">)  [unwired: 7 in]
                    n257 = call "Write.vi"("error in (no error)"=w731, "PV"=w733, "PVConnection in"=w735) -> ("error out"=w729:errorcluster)  [unwired: 7 in, 1 out]
                  }
                  event "Auto Mute": Value Change {
                    n258 = event-data() -> ("NewVal"=w744:bool)  [unwired: 1 in]
                    n259 = Index Array(array=w753, index=4) -> (element=w751:refnum<class "PVConnection.lvclass">)
                    n260 = call "Read PV.vi"("PVConnection in"=w751) -> ("error out"=w747:errorcluster, "PV"=w749:refnum<class "PV.lvclass">, "PVConnection out"=w750:refnum<class "PVConnection.lvclass">)  [unwired: 8 in]
                    n261 = call "Write Data.vi"("error in (no error)"=w747, "Data"=w744, "PV in"=w749) -> ("error out"=w746:errorcluster, "PV out"=w748:refnum<class "PV.lvclass">)  [unwired: 7 in]
                    n262 = call "Write.vi"("error in (no error)"=w746, "PV"=w748, "PVConnection in"=w750) -> ("error out"=w745:errorcluster)  [unwired: 7 in, 1 out]
                  }
                  event "Mute All": Value Change {
                    n263 = event-data() -> ("NewVal"=w759:bool)  [unwired: 1 in]
                    n264 = Index Array(array=w768, index=5) -> (element=w766:refnum<class "PVConnection.lvclass">)
                    n265 = call "Read PV.vi"("PVConnection in"=w766) -> ("error out"=w762:errorcluster, "PV"=w764:refnum<class "PV.lvclass">, "PVConnection out"=w765:refnum<class "PVConnection.lvclass">)  [unwired: 8 in]
                    n266 = call "Write Data.vi"("error in (no error)"=w762, "Data"=w759, "PV in"=w764) -> ("error out"=w761:errorcluster, "PV out"=w763:refnum<class "PV.lvclass">)  [unwired: 7 in]
                    n267 = call "Write.vi"("error in (no error)"=w761, "PV"=w763, "PVConnection in"=w765) -> ("error out"=w760:errorcluster)  [unwired: 7 in, 1 out]
                  }
                  event "Mute": Value Change {
                    n268 = event-data() -> ()  [unwired: 1 in, 1 out]
                    n269 = Index Array(array=w785, index=6) -> (element=w783:refnum<class "PVConnection.lvclass">)
                    n270 = call "Read PV.vi"("PVConnection in"=w783) -> ("error out"=w779:errorcluster, "PV"=w781:refnum<class "PV.lvclass">, "PVConnection out"=w782:refnum<class "PVConnection.lvclass">)  [unwired: 8 in]
                    n271 = Bundle("Detector"="Detector", "Mute"="Mute") -> (w776:cluster{"Detector":u8, "Mute":bool})  [unwired: 1 in]
                    n272 = call "Write Data.vi"("error in (no error)"=w779, "Data"=w776, "PV in"=w781) -> ("error out"=w778:errorcluster, "PV out"=w780:refnum<class "PV.lvclass">)  [unwired: 7 in]
                    n273 = call "Write.vi"("error in (no error)"=w778, "PV"=w780, "PVConnection in"=w782) -> ("error out"=w777:errorcluster)  [unwired: 7 in, 1 out]
                  }
                }
                "Detector Status" <- w107
                "Hardware Status" <- w106
                "Rack Status" <- w104
                "ADC Raw" <- w101
                "Voltage" <- w100
                n274 = local write "Error Out"(w110) -> ()
                n275 = disable-structure shown="Default" {
                  disable-tunnel: w110 -> [w116 _]
                  frame condition #0 (active) {
                    n276 = call <vilib>:"Simple Error Handler.vi"("error in (no error)"=w116) -> ()  [unwired: 4 in, 5 out]
                  }
                  frame condition #1 {
                  }
                }
              }
              n277 = Unregister For Events(event registration refnum=w99) -> (error out=w98:errorcluster)  [unwired: 1 in]
              n278 = call-dynamic "Destroy User Define Events.vi"("error in (no error)"=w98, "CS++GUIActor in"=w95) -> ()  [unwired: 8 in, 2 out]
            }
            frame #2 {
              n279 = call "Open Actor Core FP.vi"("Open FP (F)"=FALSE, "CS++BaseActor in"=w787) -> ()  [unwired: 8 in, 2 out]
            }
          }
        }
        frame Error {
        }
      }
    }
  }
  n280 = call-parent "Actor Core.vi"("error in"=w10, "CS++DeviceGUIActor.lvclass"=w11) -> ("Error Out"=→"Error Out":errorcluster, "Actor out"=→"Actor out":refnum<class "Actor.lvclass">)  [unwired: 8 in]
